vi "Get DDS Support Boxing Style.vi"(8 "error in (no error)":errorcluster, 11 "style":i32[](array[numeric])=[0, 0, 0, 0, 0, 0, 0, 0, 0, 0, 0, 0, 0, 0, 0, 0, 0, 0, 0, 0]) -> (0 "error out":errorcluster, 2 "function return":i32, 3 "style out":i32[](array[numeric]))   [LabVIEW 2021, in "vmmsolib.lvlib"]
doc: "DLL_API int WINAPI GetDDSSupportBoxingStyle(int* style);"
uses:
  vmmsolib.lvlib
  vmmso.dll
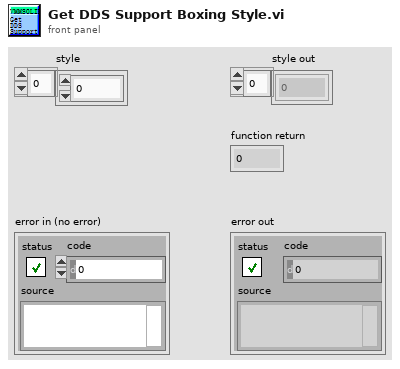
[diagram p1: front panel]
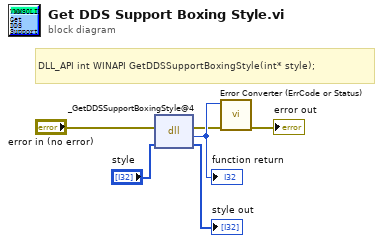
[diagram p0: block diagram]
diagram:
  # "DLL_API int WINAPI GetDDSSupportBoxingStyle(int* style);"
  n1 = dll-call lib="D:/VmMsoSDK/demo-Labview/2021/vmmsolib/vmmso.*" fn="_GetDDSSupportBoxingStyle@4"(error in="error in (no error)", "style"="style") -> (error out=w2:errorcluster, w6:i32, "style"=→"style out":i32[])  [unwired: 2 in, 1 out]
  "function return" <- w6
  n2 = call "Error Converter (ErrCode or Status).vi"("error in (no error)"=w2, "error code"=w6) -> ("error out"=→"error out":errorcluster)  [unwired: 9 in]
